vi "VRM.Get Status.vi"(6 "Axis":T1, 8 "error in (no error)":errorcluster, 11 "Instrument.VRM in":refnum<class "Instrument.OxfordVRM.lvclass">) -> (0 "error out":errorcluster, 1 "Status (ALL)":T2, 2 "Status":string[](array[string]), 3 "Instrument.VRM out":refnum<class "Instrument.OxfordVRM.lvclass">)   [LabVIEW 2019, in "Instrument.OxfordVRM.lvclass"]
doc: "Status Bits:\n[0] = Hold?\n[1] = Ramp to Set?\n[2] = Ramp to Zero?\n[3] = Clamp?"
uses:
  Instrument.OxfordVRM.lvclass
  Typedefs/VRM Magnet Axis--Enum.ctl
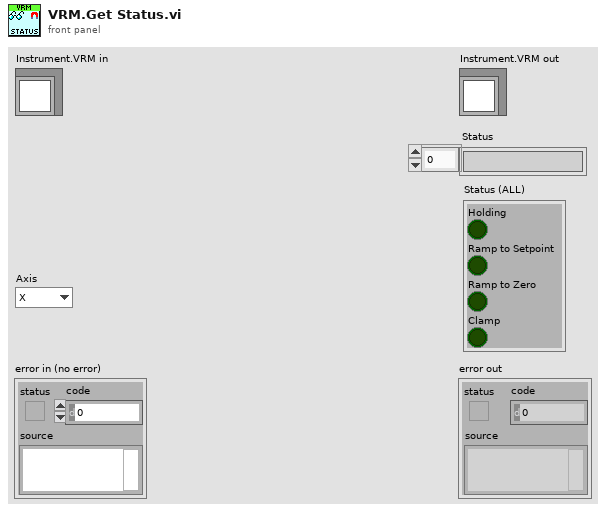
[diagram p1: front panel]
types:
  T1 = typedef "Instrument.OxfordVRM.lvclass/VRM Magnet Axis--Enum.ctl" = enum16{"X", "Y", "Z", "ALL"}
  T2 = cluster{"Holding":bool, "Ramp to Setpoint":bool, "Ramp to Zero":bool, "Clamp":bool}
  T3 = typedef "Instrument.Cryostat.lvclass/Magnet Axis--Enum.ctl" = enum16{"X", "Y", "Z"}
  T4 = cluster{"[0]":bool, "[1]":bool, "[2]":bool, "[3]":bool}
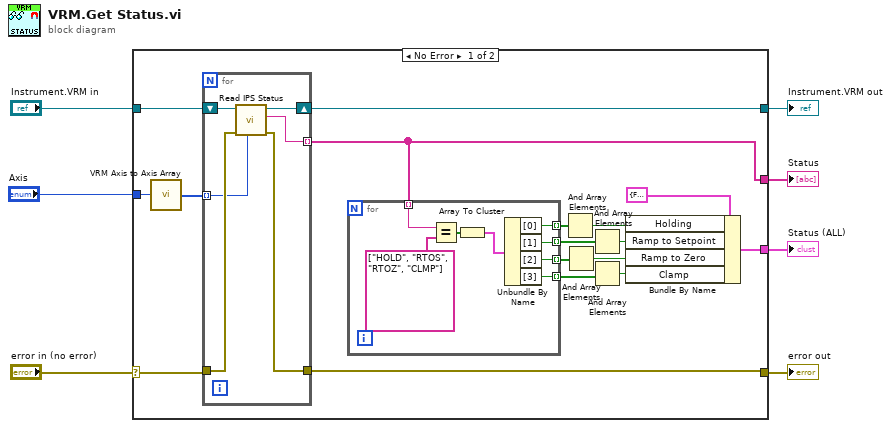
[diagram p0: block diagram]
diagram:
  n1 = case shown="No Error" "error in (no error)" {
    selector: "error in (no error)" -> [w12 w40]
    tunnel: [w11 w40] -> w6
    tunnel: [w13 w39] -> w4
    tunnel: "Instrument.VRM in" -> [w14 w39]
    tunnel: [w10 _] -> w3
    tunnel: [w15 _] -> w2
    tunnel: "Axis" -> [w9 _]
    frame No Error {
      n2 = call "VRM Axis to Axis Array.vi"("Axis"=w9) -> ("Axis Array"=w8:T3[])
      n3 = for {
        tunnel: [w26] -> w10 mode=indexing
        shift-right: [w29] -> w13
        shift-left: w14 -> [w30]
        tunnel: w8 -> [w25] mode=indexing
        tunnel: w12 -> [w28]
        tunnel: [w27] -> w11
        n4 = call "Read IPS Status.vi"("Axis"=w25, "error in (no error)"=w28, "Instrument.OxfordVRM in"=w30) -> ("error out"=w27:errorcluster, "Status"=w26:string, "Instrument.OxfordVRM out"=w29:refnum<class "Instrument.OxfordVRM.lvclass">)  [unwired: 6 in]
      }
      n5 = for {
        tunnel: w10 -> [w36] mode=indexing
        tunnel: [w34] -> w24 mode=indexing
        tunnel: [w33] -> w23 mode=indexing
        tunnel: [w32] -> w22 mode=indexing
        tunnel: [w31] -> w21 mode=indexing
        n6 = Equal?(x=w36, y=string[] ["HOLD", "RTOS", "RTOZ", "CLMP"] ("Array")) -> (x = y?=w38:bool[])
        n7 = Array To Cluster(array=w38) -> (cluster=w35:T4)
        n8 = Unbundle By Name(w35) -> ("[0]"=w34:bool, "[1]"=w33:bool, "[2]"=w32:bool, "[3]"=w31:bool)
      }
      n9 = And Array Elements(Boolean array=w24) -> (logical AND=w16:bool)
      n10 = And Array Elements(Boolean array=w22) -> (logical AND=w18:bool)
      n11 = And Array Elements(Boolean array=w23) -> (logical AND=w17:bool)
      n12 = And Array Elements(Boolean array=w21) -> (logical AND=w19:bool)
      n13 = Bundle By Name(cluster=T2 {"Holding"=FALSE, "Ramp to Setpoint"=FALSE, "Ramp to Zero"=FALSE, "Clamp"=FALSE} ("Status"), "Holding"=w16, "Ramp to Setpoint"=w17, "Ramp to Zero"=w18, "Clamp"=w19) -> (w15:T2)
    }
    frame Error {
    }
  }
  "error out" <- w6
  "Instrument.VRM out" <- w4
  "Status" <- w3
  "Status (ALL)" <- w2
